vi "Steppers_simultaneous.vi"() -> ()   [LabVIEW 2019]
uses:
  <vilib>/Instr/_visa.llb/VISA Set IO Buffer Mask.ctl
  <vilib>/Instr/_visa.llb/VISA Configure Serial Port (Instr).vi
panel:
  in  "Motor 8":i32 min=0 max=99999 format="%05.0f"
  in  "Motor 7":i32 min=0 max=99999 format="%05.0f"
  in  "Motor 6":i32 min=0 max=99999 format="%05.0f"
  in  "Motor 5":i32 min=0 max=99999 format="%05.0f"
  in  "Motor 4":i32 min=0 max=99999 format="%05.0f"
  in  "Motor 3":i32 min=0 max=99999 format="%05.0f"
  in  "Motor 2":i32 min=0 max=99999 format="%05.0f"
  in  "Motor 1":i32 min=0 max=99999 format="%05.0f"
  in  "VISA resource name":refnum<visa-resource-name>
  in  "stop":bool
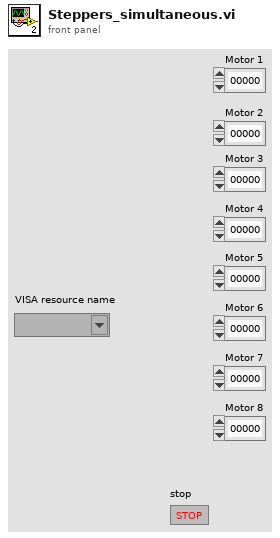
[diagram p1: front panel]
types:
  T1 = typedef "VISA Set IO Buffer Mask.ctl" = u16
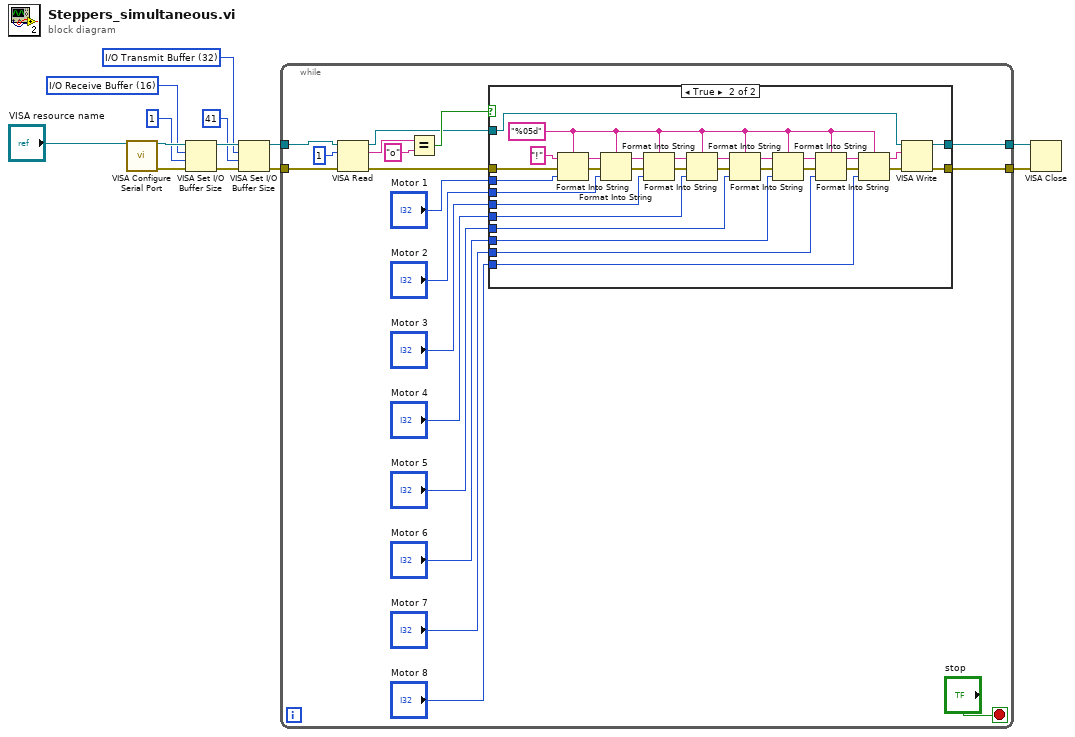
[diagram p0: block diagram]
diagram:
  w2 = T1 32 items=["I/O Receive Buffer"=16, "I/O Transmit Buffer"=32, "I/O Receive and Transmit Buffer"=48] ("Mask")
  w7 = T1 16 items=["I/O Receive Buffer"=16, "I/O Transmit Buffer"=32, "I/O Receive and Transmit Buffer"=48] ("Mask")
  n1 = call-poly "VISA Configure Serial Port"("VISA resource name"="VISA resource name") -> ("VISA resource name out"=w10:refnum<visa-resource-name>, "error out"=w9:errorcluster)  [unwired: 13 in]
  n2 = VISA Set I/O Buffer Size(VISA resource name=w10, mask (16)=w7, size (4096)=u32 1, error in (no error)=w9) -> (VISA resource name out=w5:refnum<visa-resource-name>, error out=w6:errorcluster)
  n3 = VISA Set I/O Buffer Size(VISA resource name=w5, mask (16)=w2, size (4096)=u32 41, error in (no error)=w6) -> (VISA resource name out=w4:refnum<visa-resource-name>, error out=w3:errorcluster)
  n4 = while {
    tunnel: w3 -> [w23]
    tunnel: w4 -> [w22]
    tunnel: [w24] -> w12
    tunnel: [w25] -> w11
    stop <- "stop" stop-if-true
    n5 = VISA Read(VISA resource name=w22, byte count=u32 1, error in (no error)=w23) -> (VISA resource name out=w28:refnum<visa-resource-name>, read buffer=w27:string, error out=w29:errorcluster)  [unwired: 1 out]
    n6 = Equal?(x=w27, y="o") -> (x = y?=w30:bool)
    n7 = case shown="True" w30 {
      tunnel: w28 -> [w33 w46]
      tunnel: w29 -> [w34 w43]
      tunnel: [w33 w45] -> w25
      tunnel: [w34 w44] -> w24
      tunnel: "Motor 1" -> [_ w42]
      tunnel: "Motor 2" -> [_ w41]
      tunnel: "Motor 3" -> [_ w40]
      tunnel: "Motor 4" -> [_ w39]
      tunnel: "Motor 5" -> [_ w38]
      tunnel: "Motor 6" -> [_ w37]
      tunnel: "Motor 7" -> [_ w36]
      tunnel: "Motor 8" -> [_ w35]
      frame False {
      }
      frame True {
        w48 = "%05d" ("format string")
        n8 = Format Into String(format string=w48, initial string="!" ("write buffer"), error in=w43, w42) -> (resulting string=w63:string, error out=w64:errorcluster)
        n9 = Format Into String(format string=w48, initial string=w63, error in=w64, w41) -> (resulting string=w61:string, error out=w62:errorcluster)
        n10 = Format Into String(format string=w48, initial string=w61, error in=w62, w40) -> (resulting string=w59:string, error out=w60:errorcluster)
        n11 = Format Into String(format string=w48, initial string=w59, error in=w60, w39) -> (resulting string=w57:string, error out=w58:errorcluster)
        n12 = Format Into String(format string=w48, initial string=w57, error in=w58, w38) -> (resulting string=w55:string, error out=w56:errorcluster)
        n13 = Format Into String(format string=w48, initial string=w55, error in=w56, w37) -> (resulting string=w53:string, error out=w54:errorcluster)
        n14 = Format Into String(format string=w48, initial string=w53, error in=w54, w36) -> (resulting string=w52:string, error out=w51:errorcluster)
        n15 = Format Into String(format string=w48, initial string=w52, error in=w51, w35) -> (resulting string=w49:string, error out=w50:errorcluster)
        n16 = VISA Write(VISA resource name=w46, write buffer=w49, error in (no error)=w50) -> (VISA resource name out=w45:refnum<visa-resource-name>, error out=w44:errorcluster)  [unwired: 1 out]
      }
    }
  }
  n17 = VISA Close(VISA resource name=w11, error in (no error)=w12) -> ()  [unwired: 1 out]
